vi "CameraQueryAcquire.vi"(8 "error in (no error)":errorcluster, 11 "NIvision in":refnum<class "IMAQdx.lvclass">) -> (0 "error out":errorcluster, 1 "frames_done":u32, 2 "acquiring":bool, 3 "NIvision out":refnum<class "IMAQdx.lvclass">)   [LabVIEW 2010, in "IMAQdx.lvclass"]
uses:
  IMAQdx.lvclass
  IMAQdx.lvclass/IMAQdx.ctl
  Program Files (x86)/National Instruments/LabVIEW 2010/resource/objmgr/imaqdx.rc
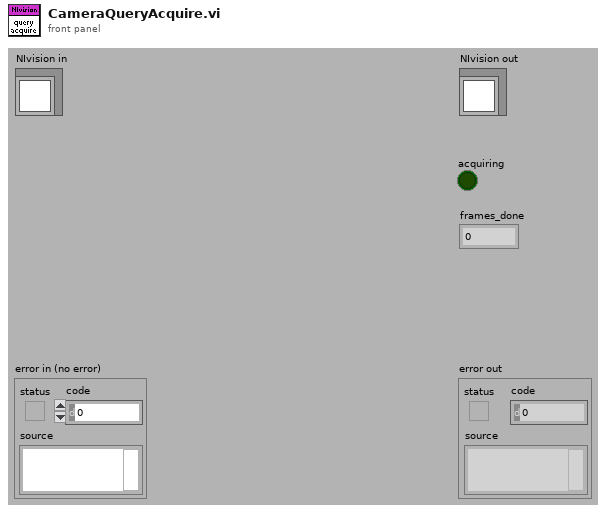
[diagram p1: front panel]
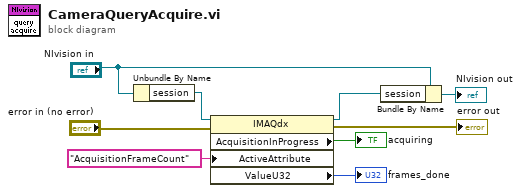
[diagram p0: block diagram]
diagram:
  n1 = Unbundle By Name("NIvision in") -> ("session"=w7:refnum<k21>)
  n2 = property class="IMAQdx"(reference=w7, error in="error in (no error)", "ActiveAttribute"="AcquisitionFrameCount") -> (reference out=w8:refnum<k21>, error out=→"error out":errorcluster, "AcquisitionInProgress"=→"acquiring":bool, "ValueU32"=→"frames_done":u32)
  n3 = Bundle By Name(cluster="NIvision in", "session"=w8) -> (→"NIvision out":refnum<class "IMAQdx.lvclass">)
